vi "LVClass_WavefrontCorrector Move to Relative Position.vi"(0 "WavefrontCorrector in":refnum<class "WavefrontCorrector.lvclass">, 5 "Wavefront Relative Position":T1, 11 "error in (no error)":errorcluster) -> (4 "WavefrontCorrector out":refnum<class "WavefrontCorrector.lvclass">, 15 "error out":errorcluster)   [LabVIEW 2020, in "WavefrontCorrector.lvclass"]
doc: "Move to requested relative positions, clip according to current preferences.\n\n--------------------------------------------------------------------------------\n\n<B>correctorIn </B> : WavefrontCorrector object.\n<B>correctorOut </B> : WavefrontCorrector object.\n<B>position </B> : Requested relatives positions.\n<B>ErrorIn </B> : Error\n<B>ErrorOut </B> : Error\n\n--------------------------------------------------------------------------------"
uses:
  WavefrontCorrector.lvclass
  Wavefront Corrector Position.ctl
  WavefrontCorrector.lvclass/WavefrontCorrector.ctl
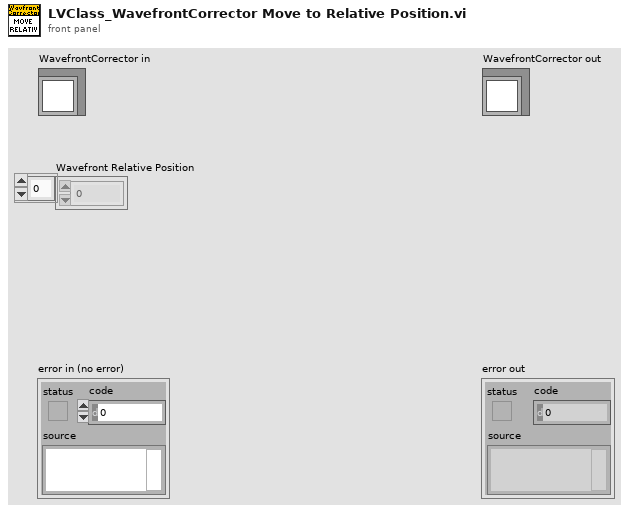
[diagram p1: front panel]
types:
  T1 = typedef "Wavefront Corrector Position.ctl" = sgl[]
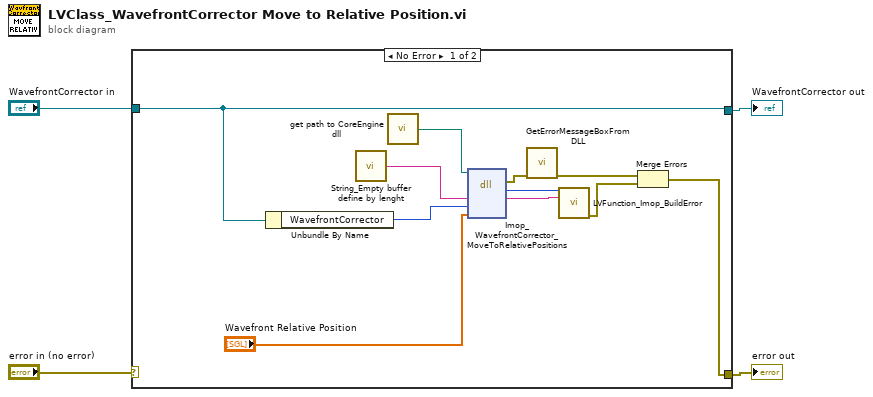
[diagram p0: block diagram]
diagram:
  n1 = case shown="No Error" "error in (no error)" {
    selector: "error in (no error)" -> [_ w17]
    tunnel: [w7 w17] -> w1
    tunnel: [w6 w16] -> w2
    tunnel: "WavefrontCorrector in" -> [w6 w16]
    frame No Error {
      n2 = Unbundle By Name(w6) -> ("WavefrontCorrector"=w8:i32)
      n3 = call "String_Empty buffer define by lenght.vi"() -> ("Empty buffer"=w13:string)  [unwired: 1 in]
      n4 = call "get path to CoreEngine dll.vi"() -> ("path to c_interface_vc100.dll"=w12:path)  [unwired: 12 in, 3 out]
      n5 = dll-call lib="D:/soft/HASO_v3/SVN_trunk/ImOpCoreEngine4_LV2011/DLLs/c_interface_vc100.dll" fn="Imop_WavefrontCorrector_MoveToRelativePositions"(path in=w12, "message"=w13, "WavefrontCorrection"=w8, "Relative Position"="Wavefront Relative Position") -> (error out=w11:errorcluster, "return type"=w15:i32, "message"=w14:string)  [unwired: 4 in, 1 out]
      n6 = call "GetErrorMessageBoxFromDLL.vi"("error IN"=w11) -> ("error OUT"=w10:errorcluster)  [unwired: 10 in]
      n7 = call "LVFunction_Imop_BuildError.vi"("code"=w15, "String to Prepend to source (\"\")"=w14) -> ("error out"=w9:errorcluster)  [unwired: 13 in]
      n8 = Merge Errors(w10, w9) -> (w7:errorcluster)
    }
    frame Error {
    }
  }
  "error out" <- w1
  "WavefrontCorrector out" <- w2
